vi "data without drive coil times in TR.vi"(0 "data":T1, 1 "buffer (s) after":dbl=0.05 format="%#_13g", 2 "t1":dbl=-1.0, 5 "coil":T1, 7 "recent interval":dbl=5.0, 9 "most recent?":bool, 11 "error in (no error)":errorcluster, 12 "buffer (s) before":dbl=-0.02 format="%#_13g", 13 "t0":dbl=-1.0) -> (4 "data_no_coil":T2[](array[typedef]), 6 "not currently in coil veto":bool, 15 "error out":errorcluster)   [LabVIEW 2017]
uses:
  typedefs/reading.ctl
  typedefs/readingType.ctl
  typedefs/reading queue.ctl
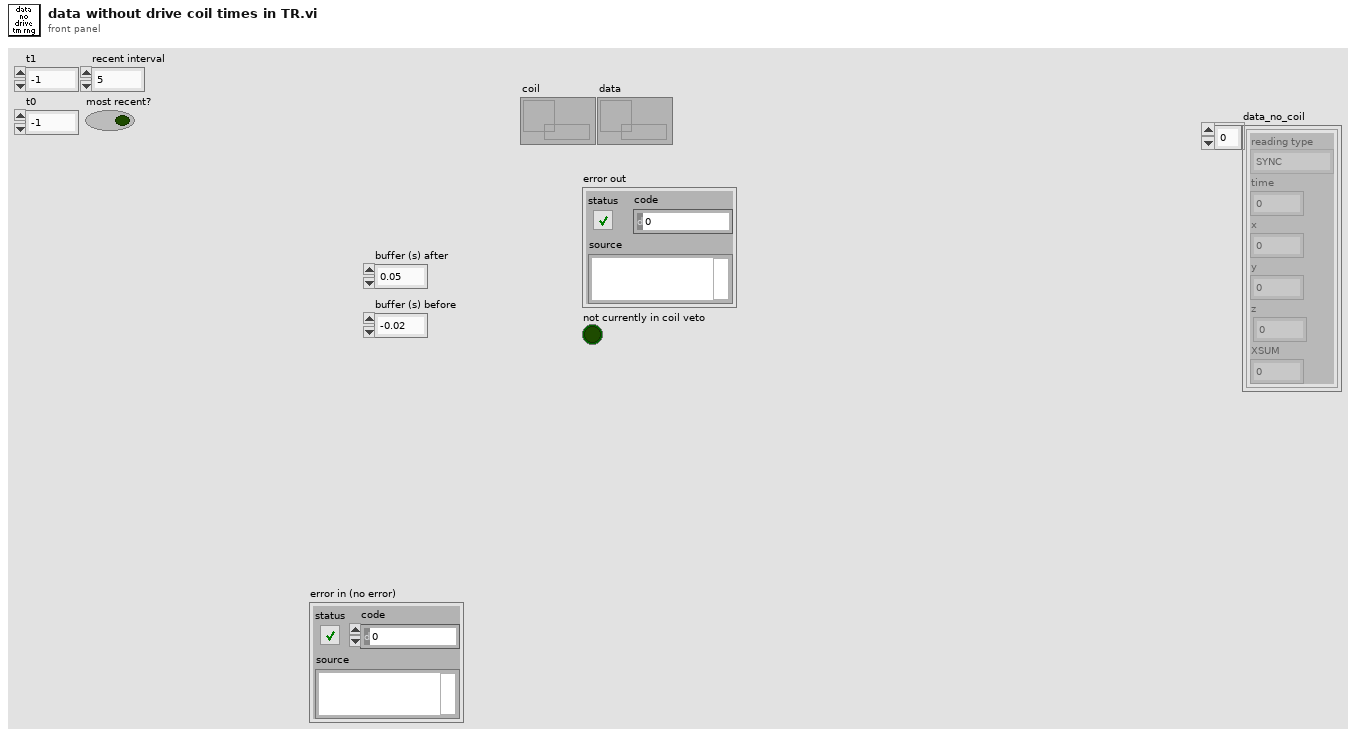
[diagram p1: front panel]
types:
  T1 = typedef "reading queue.ctl" = refnum<queue>
  T2 = typedef "reading.ctl" = cluster{"reading type":T3, "time":fxp<+,48,48>, "x":sgl, "y":sgl, "z":sgl, "XSUM":u8}
  T3 = typedef "readingType.ctl" = enum8{"SYNC", "DETVAL", "COILI", "MAGVEC", "ACCVEC"}
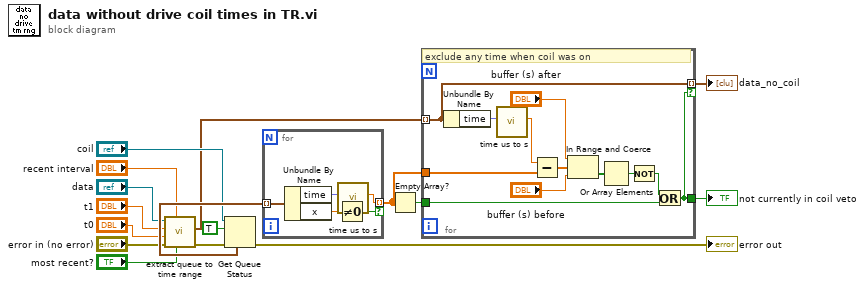
[diagram p0: block diagram]
diagram:
  n1 = call "extract queue to time range.vi"("most recent?"="most recent?", "recent interval"="recent interval", "error in (no error)"="error in (no error)", "t0"="t0", "t1"="t1", "queue"="data") -> ("error out"=w1:errorcluster, "extracted data"=w2:T2[])  [unwired: 4 in]
  n2 = Get Queue Status(queue="coil", return elements? (F)=TRUE, error in (no error)=w1) -> (error out=→"error out":errorcluster, elements=w15:T2[])  [unwired: 6 out]
  n3 = for {
    tunnel: w15 -> [w20] mode=indexing
    tunnel: [w17] -> w10 mode=indexing if=w19
    n4 = Unbundle By Name(w20) -> ("time"=w18:fxp<+,48,48>, "x"=w21:sgl)
    n5 = Not Equal To 0?(x=w21) -> (x != 0?=w19:bool)
    n6 = call "time us to s.vi"("time (us)"=w18) -> ("time (s)"=w17:dbl)  [unwired: 10 in]
  }
  n7 = Empty Array?(array=w10) -> (empty?=w9:bool)
  n8 = for {
    tunnel: w2 -> [w33] mode=indexing
    tunnel: [w33] -> w12 mode=indexing if=w24
    tunnel: w10 -> [w31]
    tunnel: [w24] -> w13
    tunnel: w9 -> [w23]
    # "exclude any time when coil was on"
    n9 = Unbundle By Name(w33) -> ("time"=w32:fxp<+,48,48>)
    n10 = call "time us to s.vi"("time (us)"=w32) -> ("time (s)"=w22:dbl)  [unwired: 10 in]
    n11 = Subtract(x=w22, y=w31) -> (x-y=w30:dbl[])
    n12 = In Range and Coerce(upper limit="buffer (s) after", x=w30, lower limit="buffer (s) before") -> (In Range?=w27:bool[])  [unwired: 1 out]
    n13 = Or Array Elements(Boolean array=w27) -> (logical OR=w26:bool)
    n14 = Not(x=w26) -> (.not. x?=w25:bool)
    n15 = Or(x=w25, y=w23) -> (x .or. y?=w24:bool)
  }
  "data_no_coil" <- w12
  "not currently in coil veto" <- w13
